vi "multiple tag creation dialog.vi"(8 "error in":errorcluster) -> (0 "error out":errorcluster, 2 "valid?":bool, 3 "new tags":refnum<class "tag descriptor.lvclass">[](array[class]))   [LabVIEW 2013, in "PL Framework Configuration Tool.lvlib" / "EngineTags.lvclass"]
uses:
  EngineTags.lvclass
  <vilib>/NI/Tag Bus/tag/tag descriptor.lvclass
  <vilib>/NI/Tag Bus/tag/tag descriptor.lvclass/tag descriptor.ctl
  <vilib>/NI/Tag Bus/tag/count types.vi
  <vilib>/NI/Tag Bus/tag/index to type.vi
  <vilib>/NI/Tag Bus/tag/default value polymorphs/write default value Double.vi
  <vilib>/NI/Tag Bus/tag/default value polymorphs/write default value Single.vi
  <vilib>/NI/Tag Bus/tag/default value polymorphs/write default value String.vi
  <vilib>/NI/Tag Bus/tag/default value polymorphs/write default value Boolean.vi
  <vilib>/NI/Tag Bus/tag/default value polymorphs/write default value Array of U8.vi
  <vilib>/NI/Tag Bus/tag/default value polymorphs/write default value Array of U16.vi
  <vilib>/NI/Tag Bus/tag/default value polymorphs/write default value Array of U32.vi
  <vilib>/NI/Tag Bus/tag/default value polymorphs/write default value Array of U64.vi
  <vilib>/NI/Tag Bus/tag/default value polymorphs/write default value Array of I64.vi
  <vilib>/NI/Tag Bus/tag/default value polymorphs/write default value Array of I32.vi
  <vilib>/NI/Tag Bus/tag/default value polymorphs/write default value Array of I16.vi
  <vilib>/NI/Tag Bus/tag/default value polymorphs/write default value Array of I8.vi
  <vilib>/NI/Tag Bus/tag/default value polymorphs/write default value Array of Double.vi
  <vilib>/NI/Tag Bus/tag/default value polymorphs/write default value Array of Single.vi
  <vilib>/NI/Tag Bus/tag/default value polymorphs/write default value Array of String.vi
  <vilib>/NI/Tag Bus/tag/default value polymorphs/write default value Array of Boolean.vi
  <vilib>/NI/Tag Bus/tag/default value polymorphs/write default value I64.vi
  <vilib>/NI/Tag Bus/tag/default value polymorphs/write default value I32.vi
  <vilib>/NI/Tag Bus/tag/default value polymorphs/write default value I16.vi
  <vilib>/NI/Tag Bus/tag/default value polymorphs/write default value I8.vi
  <vilib>/NI/Tag Bus/tag/default value polymorphs/write default value U64.vi
  <vilib>/NI/Tag Bus/tag/default value polymorphs/write default value U32.vi
  <vilib>/NI/Tag Bus/tag/default value polymorphs/write default value U16.vi
  <vilib>/NI/Tag Bus/tag/default value polymorphs/write default value U8.vi
  <vilib>/NI/Tag Bus/tag/default value polymorphs/read default value Double.vi
  <vilib>/NI/Tag Bus/tag/default value polymorphs/read default value Single.vi
  <vilib>/NI/Tag Bus/tag/default value polymorphs/read default value I64.vi
  <vilib>/NI/Tag Bus/tag/default value polymorphs/read default value I32.vi
  <vilib>/NI/Tag Bus/tag/default value polymorphs/read default value I16.vi
  <vilib>/NI/Tag Bus/tag/default value polymorphs/read default value I8.vi
  <vilib>/NI/Tag Bus/tag/default value polymorphs/read default value U64.vi
  <vilib>/NI/Tag Bus/tag/default value polymorphs/read default value U32.vi
  <vilib>/NI/Tag Bus/tag/default value polymorphs/read default value U16.vi
  <vilib>/NI/Tag Bus/tag/default value polymorphs/read default value U8.vi
  <vilib>/NI/Tag Bus/tag/default value polymorphs/read default value String.vi
  <vilib>/NI/Tag Bus/tag/default value polymorphs/read default value Boolean.vi
  <vilib>/NI/Tag Bus/tag/default value polymorphs/read default value Array of U8.vi
  <vilib>/NI/Tag Bus/tag/default value polymorphs/read default value Array of U16.vi
  <vilib>/NI/Tag Bus/tag/default value polymorphs/read default value Array of U32.vi
  <vilib>/NI/Tag Bus/tag/default value polymorphs/read default value Array of U64.vi
  <vilib>/NI/Tag Bus/tag/default value polymorphs/read default value Array of I64.vi
  <vilib>/NI/Tag Bus/tag/default value polymorphs/read default value Array of I32.vi
  <vilib>/NI/Tag Bus/tag/default value polymorphs/read default value Array of I16.vi
  <vilib>/NI/Tag Bus/tag/default value polymorphs/read default value Array of I8.vi
  <vilib>/NI/Tag Bus/tag/default value polymorphs/read default value Array of Double.vi
  <vilib>/NI/Tag Bus/tag/default value polymorphs/read default value Array of Single.vi
  <vilib>/NI/Tag Bus/tag/default value polymorphs/read default value Array of Boolean.vi
  <vilib>/NI/Tag Bus/tag/default value polymorphs/read default value Array of String.vi
panel:
  in  "Count":u16
  in  "Types":i32(listbox)
  in  "update tag":bool
  in  "Save Button":bool
  in  "numeric type":ext caption="Default Double"
  in  "string type":string
  in  "boolean type":bool
  in  "numeric array type":ext[](array[numeric])
  in  "string array type":string[](array[string])
  in  "boolean array type":bool[](array[boolean])
  in  "Tag Name":string
  in  "Tag Description":string
  in  "Cancel Button":bool
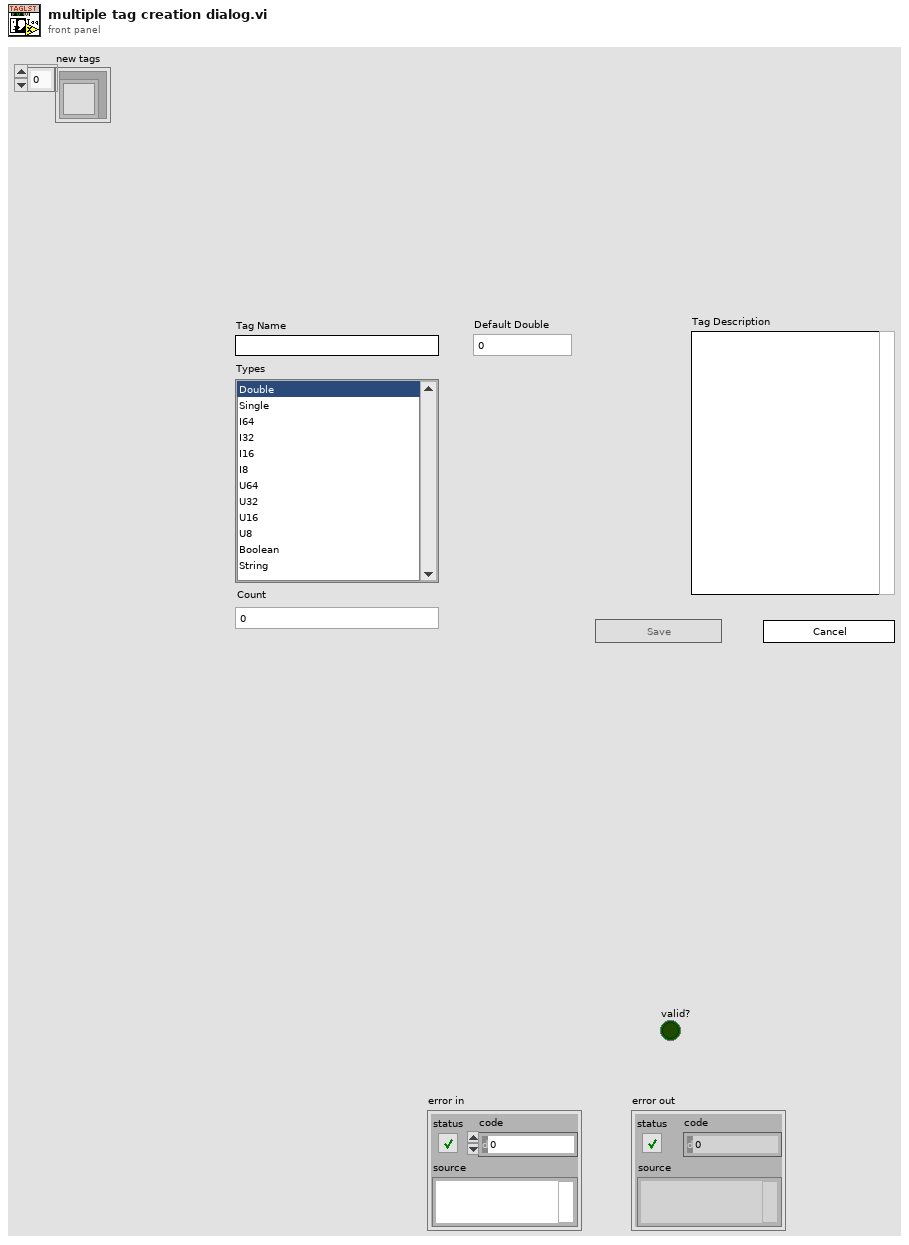
[diagram p1: front panel]
types:
  T1 = enum8{"Enabled", "Disabled", "Disabled and Grayed Out"}
  T2 = typedef "tag bus.lvlib/tag descriptor.lvclass/Data Type.ctl" = enum16{"Double", "Single", "I64", "I32", "I16", "I8", "U64", "U32", "U16", "U8", "Boolean", "String", "Array of Double", "Array of Single", "Array of I64", "Array of I32", "Array of I16", "Array of I8", "Array of U64", "Array of U32", "Array of U16", "Array of U8", "Array of Boolean", "Array of String"}
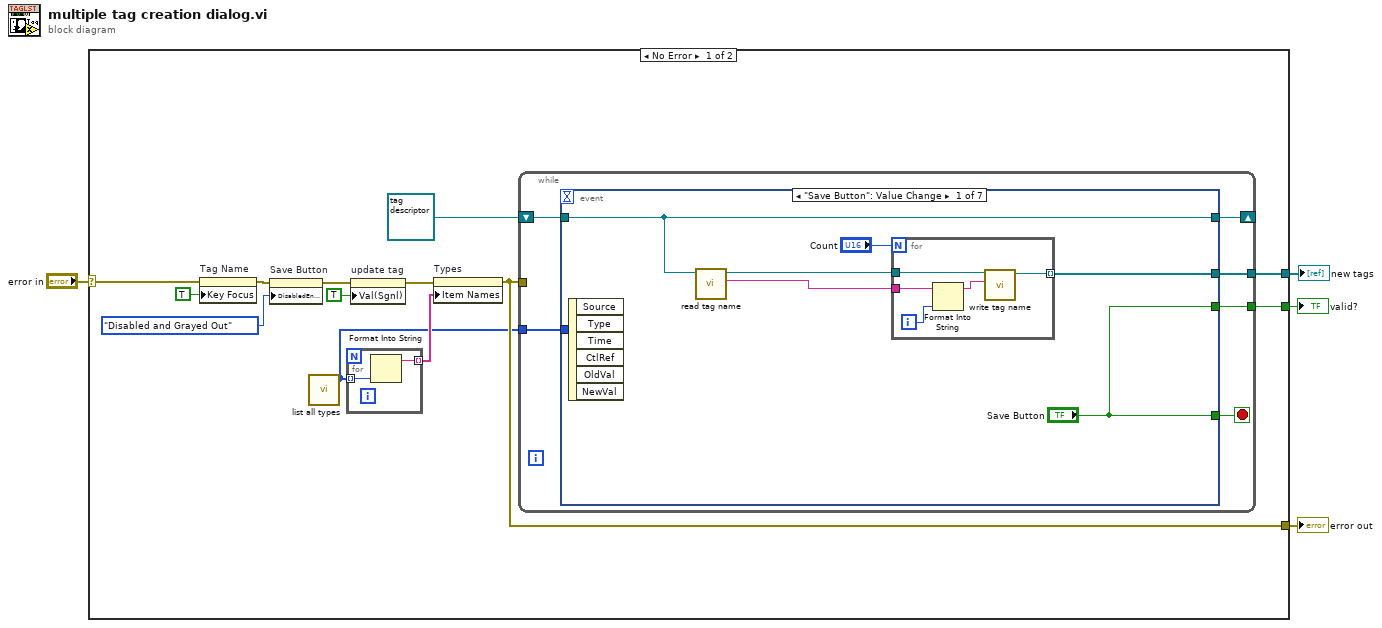
[diagram p0: block diagram]
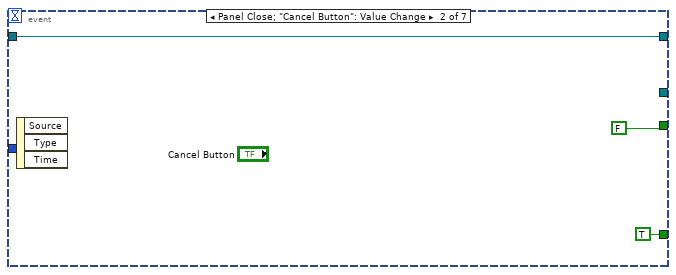
[diagram p2: hidden frame]
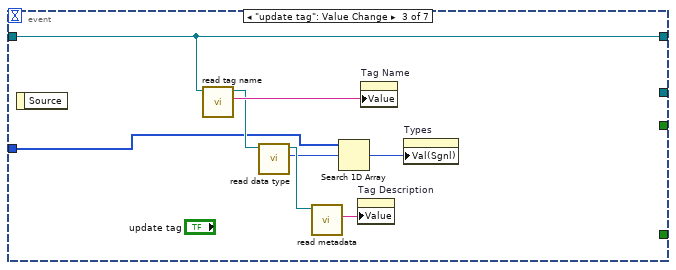
[diagram p3: hidden frame]
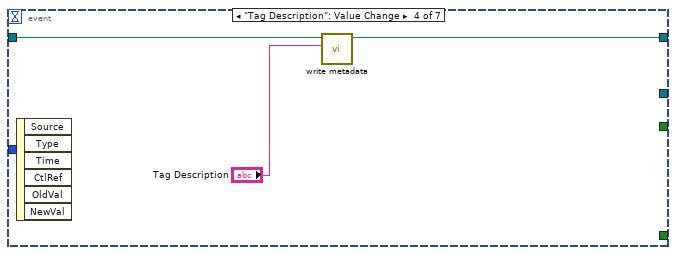
[diagram p4: hidden frame]
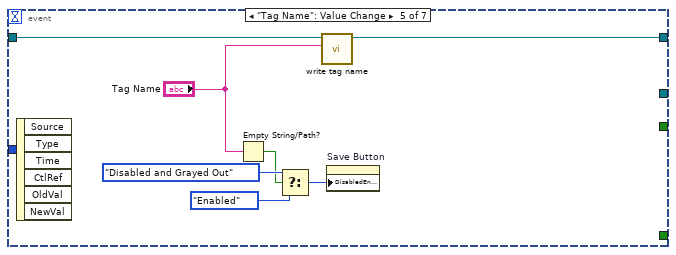
[diagram p5: hidden frame]
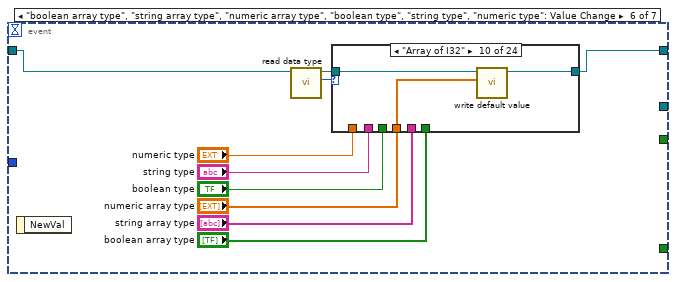
[diagram p6: hidden frame]
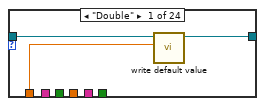
[diagram p7: hidden frame]
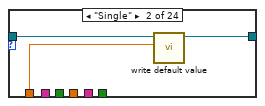
[diagram p8: hidden frame]
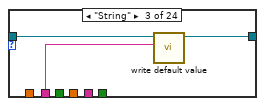
[diagram p9: hidden frame]
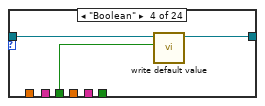
[diagram p10: hidden frame]
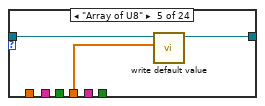
[diagram p11: hidden frame]
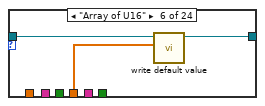
[diagram p12: hidden frame]
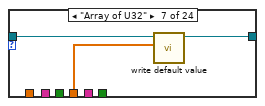
[diagram p13: hidden frame]
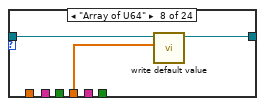
[diagram p14: hidden frame]
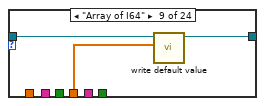
[diagram p15: hidden frame]
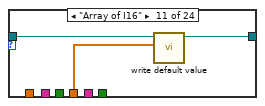
[diagram p16: hidden frame]
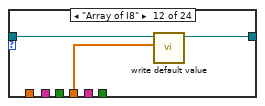
[diagram p17: hidden frame]
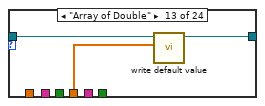
[diagram p18: hidden frame]
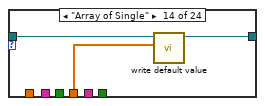
[diagram p19: hidden frame]
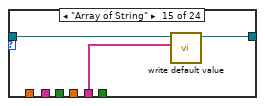
[diagram p20: hidden frame]
diagram:
  n1 = case shown="No Error" "error in" {
    selector: "error in" -> [w6 w255]
    tunnel: [w17 _] -> w4
    tunnel: [w13 w255] -> w3
    tunnel: [w8 _] -> w1
    frame No Error {
      n2 = property on="Tag Name" class="Str"(error in=w6, "Key Focus"=TRUE) -> (error out=w5:errorcluster)  [unwired: 1 in, 1 out]
      n3 = property on="Save Button" class="Bool"(error in=w5, "DisabledEnum"=T1."Disabled and Grayed Out" ("Disabled")) -> (error out=w16:errorcluster)  [unwired: 1 in, 1 out]
      n4 = call <vilib>:"list all types.vi"() -> ("all types"=w11:T2[])  [unwired: 11 in]
      n5 = for {
        tunnel: w11 -> [w19] mode=indexing
        tunnel: [w18] -> w12 mode=indexing
        n6 = Format Into String(w19) -> (resulting string=w18:string)  [unwired: 3 in, 1 out]
      }
      n7 = property on="update tag" class="Bool (strict)"(error in=w16, "Val(Sgnl)"=TRUE ("Value (Signaling)")) -> (error out=w14:errorcluster)  [unwired: 1 in, 1 out]
      n8 = property on="Types" class="LstBox (strict)"(error in=w14, "Item Names"=w12) -> (error out=w13:errorcluster)  [unwired: 1 in, 1 out]
      n9 = while {
        tunnel: [w25] -> w17
        shift-right: [w22] -> _
        shift-left: refnum<class "tag descriptor.lvclass"> refnum ("reference out") -> [w23]
        tunnel: w13 -> [_]
        tunnel: w11 -> [w21]
        tunnel: [w20] -> w8
        stop <- w24 stop-if-true
        n10 = event shown="[0] \"Save Button\": Value Change" {
          selector: _ -> [_ _ _ _ _ _ _]
          dyn-events: _ -> [_ _ _ _ _ _ _]
          timeout: _ -> [_ _ _ _ _ _ _]
          tunnel: ["Save Button" FALSE _ _ _ _ _] -> w25
          tunnel: ["Save Button" TRUE _ _ _ _ _] -> w24
          tunnel: w23 -> [w28 w37 w43 w50 w57 w59 w144]
          tunnel: [w28 w37 w43 w49 w56 w58 w143] -> w22
          tunnel: w21 -> [_ _ w41 _ _ _ w142]
          tunnel: [w29 _ _ _ _ _ _] -> w20
          event "Save Button": Value Change {
            n11 = event-data() -> ()  [unwired: 1 in, 6 out]
            n12 = call <vilib>:"read tag name.vi"("system tag in"=w28) -> ("name"=w26:string, "system tag out"=w27:refnum<class "tag descriptor.lvclass">)  [unwired: 8 in, 1 out]
            n13 = for {
              N: "Count" -> [_]
              tunnel: [w36] -> w29 mode=indexing
              tunnel: w27 -> [w35]
              tunnel: w26 -> [w33]
              i -> [w32]
              n14 = Format Into String(initial string=w33, w32) -> (resulting string=w34:string)  [unwired: 2 in, 1 out]
              n15 = call <vilib>:"write tag name.vi"("name"=w34, "system tag in"=w35) -> ("system tag out"=w36:refnum<class "tag descriptor.lvclass">)  [unwired: 8 in, 1 out]
            }
          }
          event Panel Close; "Cancel Button": Value Change {
            n16 = event-data() -> ()  [unwired: 1 in, 3 out]
          }
          event "update tag": Value Change {
            n17 = event-data() -> ()  [unwired: 1 in, 1 out]
            n18 = call <vilib>:"read tag name.vi"("system tag in"=w43) -> ("name"=w47:string, "system tag out"=w46:refnum<class "tag descriptor.lvclass">)  [unwired: 8 in, 1 out]
            n19 = call <vilib>:"read data type.vi"("system tag in"=w46) -> ("data type"=w42:T2, "system tag out"=w44:refnum<class "tag descriptor.lvclass">)  [unwired: 8 in, 1 out]
            n20 = call <vilib>:"read metadata.vi"("system tag in"=w44) -> ("metadata"=w45:string)  [unwired: 8 in, 2 out]
            n21 = Search 1D Array(1D array=w41, element=w42) -> (index of element=w40:i32)  [unwired: 1 in]
            n22 = property on="Tag Description" class="Str"("Value"=w45) -> ()  [unwired: 2 in, 2 out]
            n23 = property on="Tag Name" class="Str"("Value"=w47) -> ()  [unwired: 2 in, 2 out]
            n24 = property on="Types" class="LstBox (strict)"("Val(Sgnl)"=w40) -> ()  [unwired: 2 in, 2 out]
          }
          event "Tag Description": Value Change {
            n25 = event-data() -> ()  [unwired: 1 in, 6 out]
            n26 = call <vilib>:"write metadata.vi"("metadata"="Tag Description", "system tag in"=w50) -> ("system tag out"=w49:refnum<class "tag descriptor.lvclass">)  [unwired: 8 in, 1 out]
          }
          event "Tag Name": Value Change {
            n27 = event-data() -> ()  [unwired: 1 in, 6 out]
            n28 = Empty String/Path?(string/path="Tag Name") -> (empty?=w53:bool)
            n29 = Select(t=T1."Disabled and Grayed Out" ("Disabled"), s=w53, f=T1."Enabled") -> (s? t:f=w52:T1)
            n30 = call <vilib>:"write tag name.vi"("name"="Tag Name", "system tag in"=w57) -> ("system tag out"=w56:refnum<class "tag descriptor.lvclass">)  [unwired: 8 in, 1 out]
            n31 = property on="Save Button" class="Bool"("DisabledEnum"=w52) -> ()  [unwired: 2 in, 2 out]
          }
          event "boolean array type", "string array type", "numeric array type", "boolean type", "string type", "numeric type": Value Change {
            n32 = event-data() -> ()  [unwired: 1 in, 1 out]
            n33 = call <vilib>:"read data type.vi"("system tag in"=w59) -> ("data type"=w60:T2, "system tag out"=w61:refnum<class "tag descriptor.lvclass">)  [unwired: 8 in, 1 out]
            n34 = case shown="\"Array of I32\"" w60 {
              tunnel: [w70 w73 w76 w79 w82 w85 w88 w91 w94 w97 w100 w103 w106 w109 w112 w115 w118 w121 w124 w127 w130 w133 w136 w139] -> w58
              tunnel: w61 -> [w69 w72 w75 w78 w81 w84 w87 w90 w93 w96 w99 w102 w105 w108 w111 w114 w117 w120 w123 w126 w129 w132 w135 w138]
              tunnel: "numeric type" -> [w68 w71 _ _ _ _ _ _ _ _ _ _ _ _ _ _ w116 w119 w122 w125 w128 w131 w134 w137]
              tunnel: "string type" -> [_ _ w74 _ _ _ _ _ _ _ _ _ _ _ _ _ _ _ _ _ _ _ _ _]
              tunnel: "boolean type" -> [_ _ _ w77 _ _ _ _ _ _ _ _ _ _ _ _ _ _ _ _ _ _ _ _]
              tunnel: "numeric array type" -> [_ _ _ _ w80 w83 w86 w89 w92 w95 w98 w101 w104 w107 _ _ _ _ _ _ _ _ _ _]
              tunnel: "string array type" -> [_ _ _ _ _ _ _ _ _ _ _ _ _ _ w110 _ _ _ _ _ _ _ _ _]
              tunnel: "boolean array type" -> [_ _ _ _ _ _ _ _ _ _ _ _ _ _ _ w113 _ _ _ _ _ _ _ _]
              frame "Double" {
                n35 = call-poly <vilib>:"write default value.vi"("default value"=w68, "system tag in"=w69) -> ("system tag out"=w70:refnum<class "tag descriptor.lvclass">)  [unwired: 8 in, 1 out]
              }
              frame "Single" {
                n36 = call-poly <vilib>:"write default value.vi"("default value"=w71, "system tag in"=w72) -> ("system tag out"=w73:refnum<class "tag descriptor.lvclass">)  [unwired: 8 in, 1 out]
              }
              frame "String" {
                n37 = call-poly <vilib>:"write default value.vi"("default value"=w74, "system tag in"=w75) -> ("system tag out"=w76:refnum<class "tag descriptor.lvclass">)  [unwired: 8 in, 1 out]
              }
              frame "Boolean" {
                n38 = call-poly <vilib>:"write default value.vi"("default value"=w77, "system tag in"=w78) -> ("system tag out"=w79:refnum<class "tag descriptor.lvclass">)  [unwired: 8 in, 1 out]
              }
              frame "Array of U8" {
                n39 = call-poly <vilib>:"write default value.vi"("default value"=w80, "system tag in"=w81) -> ("system tag out"=w82:refnum<class "tag descriptor.lvclass">)  [unwired: 8 in, 1 out]
              }
              frame "Array of U16" {
                n40 = call-poly <vilib>:"write default value.vi"("default value"=w83, "system tag in"=w84) -> ("system tag out"=w85:refnum<class "tag descriptor.lvclass">)  [unwired: 8 in, 1 out]
              }
              frame "Array of U32" {
                n41 = call-poly <vilib>:"write default value.vi"("default value"=w86, "system tag in"=w87) -> ("system tag out"=w88:refnum<class "tag descriptor.lvclass">)  [unwired: 8 in, 1 out]
              }
              frame "Array of U64" {
                n42 = call-poly <vilib>:"write default value.vi"("default value"=w89, "system tag in"=w90) -> ("system tag out"=w91:refnum<class "tag descriptor.lvclass">)  [unwired: 8 in, 1 out]
              }
              frame "Array of I64" {
                n43 = call-poly <vilib>:"write default value.vi"("default value"=w92, "system tag in"=w93) -> ("system tag out"=w94:refnum<class "tag descriptor.lvclass">)  [unwired: 8 in, 1 out]
              }
              frame "Array of I32" {
                n44 = call-poly <vilib>:"write default value.vi"("default value"=w95, "system tag in"=w96) -> ("system tag out"=w97:refnum<class "tag descriptor.lvclass">)  [unwired: 8 in, 1 out]
              }
              frame "Array of I16" {
                n45 = call-poly <vilib>:"write default value.vi"("default value"=w98, "system tag in"=w99) -> ("system tag out"=w100:refnum<class "tag descriptor.lvclass">)  [unwired: 8 in, 1 out]
              }
              frame "Array of I8" {
                n46 = call-poly <vilib>:"write default value.vi"("default value"=w101, "system tag in"=w102) -> ("system tag out"=w103:refnum<class "tag descriptor.lvclass">)  [unwired: 8 in, 1 out]
              }
              frame "Array of Double" {
                n47 = call-poly <vilib>:"write default value.vi"("default value"=w104, "system tag in"=w105) -> ("system tag out"=w106:refnum<class "tag descriptor.lvclass">)  [unwired: 8 in, 1 out]
              }
              frame "Array of Single" {
                n48 = call-poly <vilib>:"write default value.vi"("default value"=w107, "system tag in"=w108) -> ("system tag out"=w109:refnum<class "tag descriptor.lvclass">)  [unwired: 8 in, 1 out]
              }
              frame "Array of String" {
                n49 = call-poly <vilib>:"write default value.vi"("default value"=w110, "system tag in"=w111) -> ("system tag out"=w112:refnum<class "tag descriptor.lvclass">)  [unwired: 8 in, 1 out]
              }
              frame "Array of Boolean" {
                n50 = call-poly <vilib>:"write default value.vi"("default value"=w113, "system tag in"=w114) -> ("system tag out"=w115:refnum<class "tag descriptor.lvclass">)  [unwired: 8 in, 1 out]
              }
              frame "I64" {
                n51 = call-poly <vilib>:"write default value.vi"("default value"=w116, "system tag in"=w117) -> ("system tag out"=w118:refnum<class "tag descriptor.lvclass">)  [unwired: 8 in, 1 out]
              }
              frame "I32" {
                n52 = call-poly <vilib>:"write default value.vi"("default value"=w119, "system tag in"=w120) -> ("system tag out"=w121:refnum<class "tag descriptor.lvclass">)  [unwired: 8 in, 1 out]
              }
              frame "I16" {
                n53 = call-poly <vilib>:"write default value.vi"("default value"=w122, "system tag in"=w123) -> ("system tag out"=w124:refnum<class "tag descriptor.lvclass">)  [unwired: 8 in, 1 out]
              }
              frame "I8" {
                n54 = call-poly <vilib>:"write default value.vi"("default value"=w125, "system tag in"=w126) -> ("system tag out"=w127:refnum<class "tag descriptor.lvclass">)  [unwired: 8 in, 1 out]
              }
              frame "U64" {
                n55 = call-poly <vilib>:"write default value.vi"("default value"=w128, "system tag in"=w129) -> ("system tag out"=w130:refnum<class "tag descriptor.lvclass">)  [unwired: 8 in, 1 out]
              }
              frame "U32" {
                n56 = call-poly <vilib>:"write default value.vi"("default value"=w131, "system tag in"=w132) -> ("system tag out"=w133:refnum<class "tag descriptor.lvclass">)  [unwired: 8 in, 1 out]
              }
              frame "U16" {
                n57 = call-poly <vilib>:"write default value.vi"("default value"=w134, "system tag in"=w135) -> ("system tag out"=w136:refnum<class "tag descriptor.lvclass">)  [unwired: 8 in, 1 out]
              }
              frame "U8" {
                n58 = call-poly <vilib>:"write default value.vi"("default value"=w137, "system tag in"=w138) -> ("system tag out"=w139:refnum<class "tag descriptor.lvclass">)  [unwired: 8 in, 1 out]
              }
            }
          }
          event "Types": Value Change {
            n59 = event-data() -> ()  [unwired: 1 in, 6 out]
            n60 = Index Array(array=w142, index="Types") -> (element=w140:T2)
            n61 = control-ref of="boolean type"() -> (w153:refnum<vi>)
            n62 = control-ref of="numeric type"() -> (w151:refnum<vi>)
            n63 = control-ref of="string type"() -> (w152:refnum<vi>)
            n64 = control-ref of="boolean array type"() -> (w150:refnum<vi>)
            n65 = control-ref of="string array type"() -> (w149:refnum<vi>)
            n66 = control-ref of="numeric array type"() -> (w148:refnum<vi>)
            n67 = Build Array(w153, w152, w151, w150, w149, w148) -> (w147:refnum<vi>[])
            n68 = call <vilib>:"write data type.vi"("data type"=w140, "system tag in"=w144) -> ("system tag out"=w146:refnum<class "tag descriptor.lvclass">)  [unwired: 8 in, 1 out]
            n69 = for {
              tunnel: w147 -> [w254] mode=indexing
              tunnel: [w252] -> w145
              n70 = property class="Ctl"(reference=w254, "Visible"=FALSE) -> (error out=w252:errorcluster)  [unwired: 1 in, 1 out]
            }
            n71 = case shown="\"Array of Double\"..\"Array of U8\"" w140 {
              selector: w140 -> [w154 _ _ w203 _ _]
              tunnel: w146 -> [w157 w195 w200 w206 w244 w249]
              tunnel: [w156 w194 w199 w205 w243 w247] -> w143
              tunnel: w145 -> [_ _ _ _ _ _]
              frame "Double".."U8" {
                n72 = case shown="\"Single\"" w154 {
                  tunnel: w157 -> [w162 w165 w168 w171 w174 w177 w180 w183 w186 w189 w192]
                  tunnel: [w162 w164 w167 w170 w173 w176 w179 w182 w185 w188 w191] -> w156
                  tunnel: [ext 0.0 ("default value") w163 w166 w169 w172 w175 w178 w181 w184 w187 w190] -> w155
                  frame Default {
                  }
                  frame "Double" {
                    n73 = call-poly <vilib>:"read default value.vi"("system tag in"=w165) -> ("default value"=w163:dbl, "system tag out"=w164:refnum<class "tag descriptor.lvclass">)  [unwired: 7 in, 2 out]
                  }
                  frame "Single" {
                    n74 = call-poly <vilib>:"read default value.vi"("system tag in"=w168) -> ("default value"=w166:sgl, "system tag out"=w167:refnum<class "tag descriptor.lvclass">)  [unwired: 7 in, 2 out]
                  }
                  frame "I64" {
                    n75 = call-poly <vilib>:"read default value.vi"("system tag in"=w171) -> ("default value"=w169:i64, "system tag out"=w170:refnum<class "tag descriptor.lvclass">)  [unwired: 7 in, 2 out]
                  }
                  frame "I32" {
                    n76 = call-poly <vilib>:"read default value.vi"("system tag in"=w174) -> ("default value"=w172:i32, "system tag out"=w173:refnum<class "tag descriptor.lvclass">)  [unwired: 7 in, 2 out]
                  }
                  frame "I16" {
                    n77 = call-poly <vilib>:"read default value.vi"("system tag in"=w177) -> ("default value"=w175:i16, "system tag out"=w176:refnum<class "tag descriptor.lvclass">)  [unwired: 7 in, 2 out]
                  }
                  frame "I8" {
                    n78 = call-poly <vilib>:"read default value.vi"("system tag in"=w180) -> ("default value"=w178:i8, "system tag out"=w179:refnum<class "tag descriptor.lvclass">)  [unwired: 7 in, 2 out]
                  }
                  frame "U64" {
                    n79 = call-poly <vilib>:"read default value.vi"("system tag in"=w183) -> ("default value"=w181:u64, "system tag out"=w182:refnum<class "tag descriptor.lvclass">)  [unwired: 7 in, 2 out]
                  }
                  frame "U32" {
                    n80 = call-poly <vilib>:"read default value.vi"("system tag in"=w186) -> ("default value"=w184:u32, "system tag out"=w185:refnum<class "tag descriptor.lvclass">)  [unwired: 7 in, 2 out]
                  }
                  frame "U16" {
                    n81 = call-poly <vilib>:"read default value.vi"("system tag in"=w189) -> ("default value"=w187:u16, "system tag out"=w188:refnum<class "tag descriptor.lvclass">)  [unwired: 7 in, 2 out]
                  }
                  frame "U8" {
                    n82 = call-poly <vilib>:"read default value.vi"("system tag in"=w192) -> ("default value"=w190:u8, "system tag out"=w191:refnum<class "tag descriptor.lvclass">)  [unwired: 7 in, 2 out]
                  }
                }
                n83 = Format Into String(format string="Default %s", w154) -> (resulting string=w159:string)  [unwired: 2 in, 1 out]
                n84 = property on="numeric type" class="DigNum (strict)"("Val(Sgnl)"=w155, "Visible"=TRUE, "Caption.Text"=w159) -> ()  [unwired: 2 in, 2 out]
              }
              frame "String" {
                n85 = call-poly <vilib>:"read default value.vi"("system tag in"=w195) -> ("default value"=w193:string, "system tag out"=w194:refnum<class "tag descriptor.lvclass">)  [unwired: 7 in, 2 out]
                n86 = property on="string type" class="Str"("Val(Sgnl)"=w193, "Visible"=TRUE, "Caption.Text"="Default string" ("format string")) -> ()  [unwired: 2 in, 2 out]
              }
              frame "Boolean" {
                n87 = call-poly <vilib>:"read default value.vi"("system tag in"=w200) -> ("default value"=w198:bool, "system tag out"=w199:refnum<class "tag descriptor.lvclass">)  [unwired: 7 in, 2 out]
                n88 = property on="boolean type" class="Bool (strict)"("Val(Sgnl)"=w198, "Visible"=TRUE, "Caption.Text"="Default booleans" ("format string")) -> ()  [unwired: 2 in, 2 out]
              }
              frame "Array of Double".."Array of U8" {
                n89 = case shown="\"Array of U64\"" w203 {
                  tunnel: w206 -> [w211 w214 w217 w220 w223 w226 w229 w232 w235 w238 w241]
                  tunnel: [w211 w213 w216 w219 w222 w225 w228 w231 w234 w237 w240] -> w205
                  tunnel: [ext[] [] ("default value") w212 w215 w218 w221 w224 w227 w230 w233 w236 w239] -> w204
                  frame Default {
                  }
                  frame "Array of U8" {
                    n90 = call-poly <vilib>:"read default value.vi"("system tag in"=w214) -> ("default value"=w212:u8[], "system tag out"=w213:refnum<class "tag descriptor.lvclass">)  [unwired: 7 in, 2 out]
                  }
                  frame "Array of U16" {
                    n91 = call-poly <vilib>:"read default value.vi"("system tag in"=w217) -> ("default value"=w215:u16[], "system tag out"=w216:refnum<class "tag descriptor.lvclass">)  [unwired: 7 in, 2 out]
                  }
                  frame "Array of U32" {
                    n92 = call-poly <vilib>:"read default value.vi"("system tag in"=w220) -> ("default value"=w218:u32[], "system tag out"=w219:refnum<class "tag descriptor.lvclass">)  [unwired: 7 in, 2 out]
                  }
                  frame "Array of U64" {
                    n93 = call-poly <vilib>:"read default value.vi"("system tag in"=w223) -> ("default value"=w221:u64[], "system tag out"=w222:refnum<class "tag descriptor.lvclass">)  [unwired: 7 in, 2 out]
                  }
                  frame "Array of I64" {
                    n94 = call-poly <vilib>:"read default value.vi"("system tag in"=w226) -> ("default value"=w224:i64[], "system tag out"=w225:refnum<class "tag descriptor.lvclass">)  [unwired: 7 in, 2 out]
                  }
                  frame "Array of I32" {
                    n95 = call-poly <vilib>:"read default value.vi"("system tag in"=w229) -> ("default value"=w227:i32[], "system tag out"=w228:refnum<class "tag descriptor.lvclass">)  [unwired: 7 in, 2 out]
                  }
                  frame "Array of I16" {
                    n96 = call-poly <vilib>:"read default value.vi"("system tag in"=w232) -> ("default value"=w230:i16[], "system tag out"=w231:refnum<class "tag descriptor.lvclass">)  [unwired: 7 in, 2 out]
                  }
                  frame "Array of I8" {
                    n97 = call-poly <vilib>:"read default value.vi"("system tag in"=w235) -> ("default value"=w233:i8[], "system tag out"=w234:refnum<class "tag descriptor.lvclass">)  [unwired: 7 in, 2 out]
                  }
                  frame "Array of Double" {
                    n98 = call-poly <vilib>:"read default value.vi"("system tag in"=w238) -> ("default value"=w236:dbl[], "system tag out"=w237:refnum<class "tag descriptor.lvclass">)  [unwired: 7 in, 2 out]
                  }
                  frame "Array of Single" {
                    n99 = call-poly <vilib>:"read default value.vi"("system tag in"=w241) -> ("default value"=w239:sgl[], "system tag out"=w240:refnum<class "tag descriptor.lvclass">)  [unwired: 7 in, 2 out]
                  }
                }
                n100 = Format Into String(format string="Default %ss", w203) -> (resulting string=w208:string)  [unwired: 2 in, 1 out]
                n101 = property on="numeric array type" class="Arr (strict)"("Val(Sgnl)"=w204, "Visible"=TRUE, "Caption.Text"=w208) -> ()  [unwired: 2 in, 2 out]
              }
              frame "Array of Boolean" {
                n102 = call-poly <vilib>:"read default value.vi"("system tag in"=w244) -> ("default value"=w242:bool[], "system tag out"=w243:refnum<class "tag descriptor.lvclass">)  [unwired: 7 in, 2 out]
                n103 = property on="boolean array type" class="Arr (strict)"("Val(Sgnl)"=w242, "Visible"=TRUE, "Caption.Text"="Default booleans") -> ()  [unwired: 2 in, 2 out]
              }
              frame "Array of String" {
                n104 = call-poly <vilib>:"read default value.vi"("system tag in"=w249) -> ("default value"=w248:string[], "system tag out"=w247:refnum<class "tag descriptor.lvclass">)  [unwired: 7 in, 2 out]
                n105 = property on="string array type" class="Arr (strict)"("Val(Sgnl)"=w248, "Visible"=TRUE, "Caption.Text"="Default strings") -> ()  [unwired: 2 in, 2 out]
              }
            }
          }
        }
      }
    }
    frame Error {
    }
  }
  "error out" <- w3
  "valid?" <- w4
  "new tags" <- w1
